vi "两路模拟量输入.vi"(8 "第2路值":sgl format="%.2f", 9 "选择第2路？":bool, 10 "第1路值":sgl format="%.2f", 11 "选择第1路？":bool) -> ()   [LabVIEW 2010]
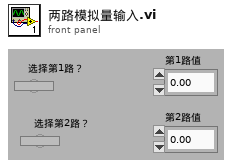
[diagram p1: front panel]
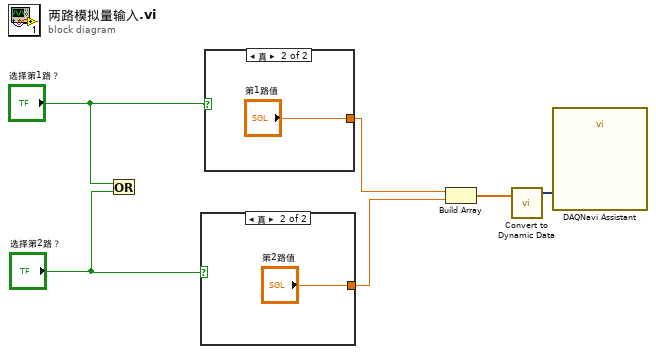
[diagram p0: block diagram]
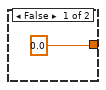
[diagram p2: hidden frame]
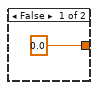
[diagram p3: hidden frame]
diagram:
  n1 = Or(x="选择第1路？", y="选择第2路？") -> (x .or. y?=w7:bool)
  n2 = case shown="真" "选择第2路？" {
    tunnel: [sgl 0.0 "第2路值"] -> w2
    frame False {
    }
    frame True {
    }
  }
  n3 = case shown="真" "选择第1路？" {
    tunnel: [sgl 0.0 "第1路值"] -> w3
    frame False {
    }
    frame True {
    }
  }
  n4 = Build Array(w3, w2) -> (w1:sgl[])
  n5 = call "Convert to Dynamic Data"("Array"=w1) -> ("Dynamic Data Type"=w4:dynamicdata)  [unwired: 3 out]
  n6 = call "DAQNavi Assistant"("data in(DDT)"=w4) -> ()  [unwired: 2 in, 17 out]
